vi "Proyecto 1.vi"() -> ()   [LabVIEW 2020]
uses:
  <vilib>/numeric/Random Number (Range) U64.vi
  <vilib>/numeric/Random Number (Range) I64.vi
  <vilib>/numeric/sub_Random U32.vi
panel:
  out "enum5":i16
  out "sum":i16
  out "Enum 4":enum8{"0", "1", "2", "3", "4", "5", "6"}(ring)
  out "Enum 3":enum8{"1", "2", "3", "4", "5", "6"}(ring)
  out "DiskAcum":i64
  out "TAP 2":string[][](array[string])
  out "Size":string[](array[string])
  out "MemoryMap":string[](array[string])
  out "TAP":string[][](array[string])
  out "Waiting 2":string[](array[string])
  out "Printing 2":string
  in  "FrameSize":i8(slide) step=1 scale=4.0..64.0
  in  "RAMSize":i64(slide) min=0 step=4 scale=32.0..256.0
  in  "ProbMemoria":i8(slide) step=10 scale=0.0..100.0
  out "element":string
  out "ID":string[](array[string])
  out "QuantumAcum":i64
  out "Enum 2":enum16{"1", "2", "3"}(ring)
  out "Tiempo de impresión":string[](array[string])
  out "Hora uso i/o":string[](array[string])
  out "Uso de impresora":string[](array[string])
  out "Duración":string[](array[string])
  out "Enum":enum16{"1", "2", "3"}(ring)=enum."3"
  out "Hora de llegada":string[](array[string])
  out "PCB":string[][](array[string])
  out "Terminated":string[](array[string])
  out "Waiting":string[](array[string])
  out "Ready":string[](array[string])
  out "New":string[](array[string])
  out "Printing":string
  out "Running":string
  in  "Delay":i32(slide)
  out "Clock":i32
  in  "play/pause":bool
  in  "DurImpresora":i8(slide) step=10 scale=10.0..80.0
  in  "ProbImpresora":i8(slide) step=10 scale=0.0..100.0
  in  "DurProceso":i8(slide) step=10 scale=5.0..100.0
  in  "Quantum":i8(slide) step=10 scale=0.0..20.0
  in  "stop":bool
  in  "ProbProceso":i8(slide) step=10 scale=0.0..100.0
  # "RELOJ"
  # "PROCESS & MEMORY MANAGER"
  # "LENTO"
  # "NORMAL"
  # "RÁPIDO"
  # "QUANTUM"
  # "NEW"
  # "READY"
  # "RUNNING"
  # "WAITING I/0"
  # "USING I/0"
  # "WAITING DISK"
  # "USING DISK"
  # "TERMINATED"
  # "MEMORY MAP"
  # "0\n1\n2\n3\n4\n5\n6\n7\n8\n9\n10\n11\n12\n13\n14\n15\n16\n17\n18\n19\n20\n21\n22\n23\n24"
  # "PROB GENERAR PROCESO"
  # "DURACIÓN PROCESO"
  # "PROB USO I/0"
  # "TAP"
  # "PROCESS CONTROL BLOCK"
  # "e"
  # "d"
  # "H I/O"
  # "ID"
  # "a"
  # "b"
  # "c"
  # "f"
  # "I/O"
  # "T I/O"
  # "SIZE (KB)"
  # "ID"
  # "AT"
  # "DUR"
  # "ACUM"
  # "DURACIÓN I/0"
  # "PROB USO MEMORIA"
  # "RAM SIZE"
  # "FRAME SIZE"
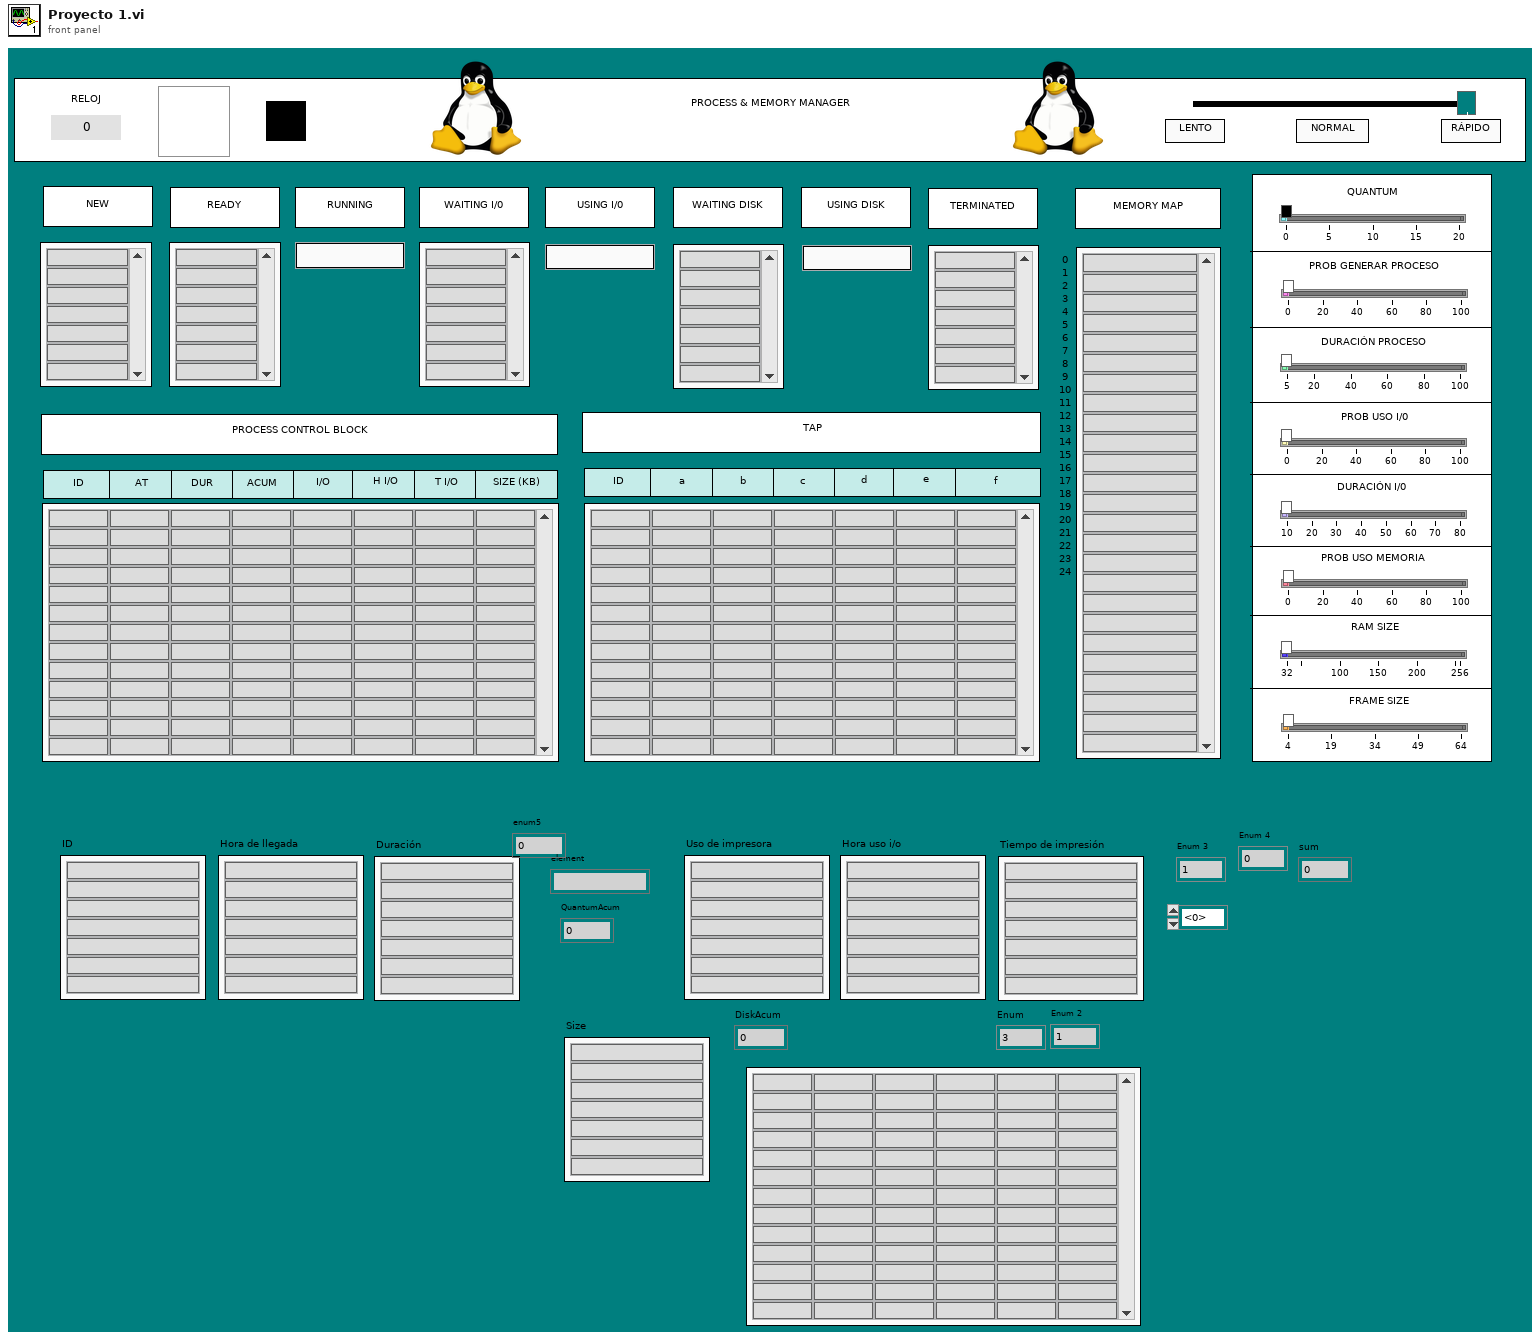
[diagram p1: front panel]
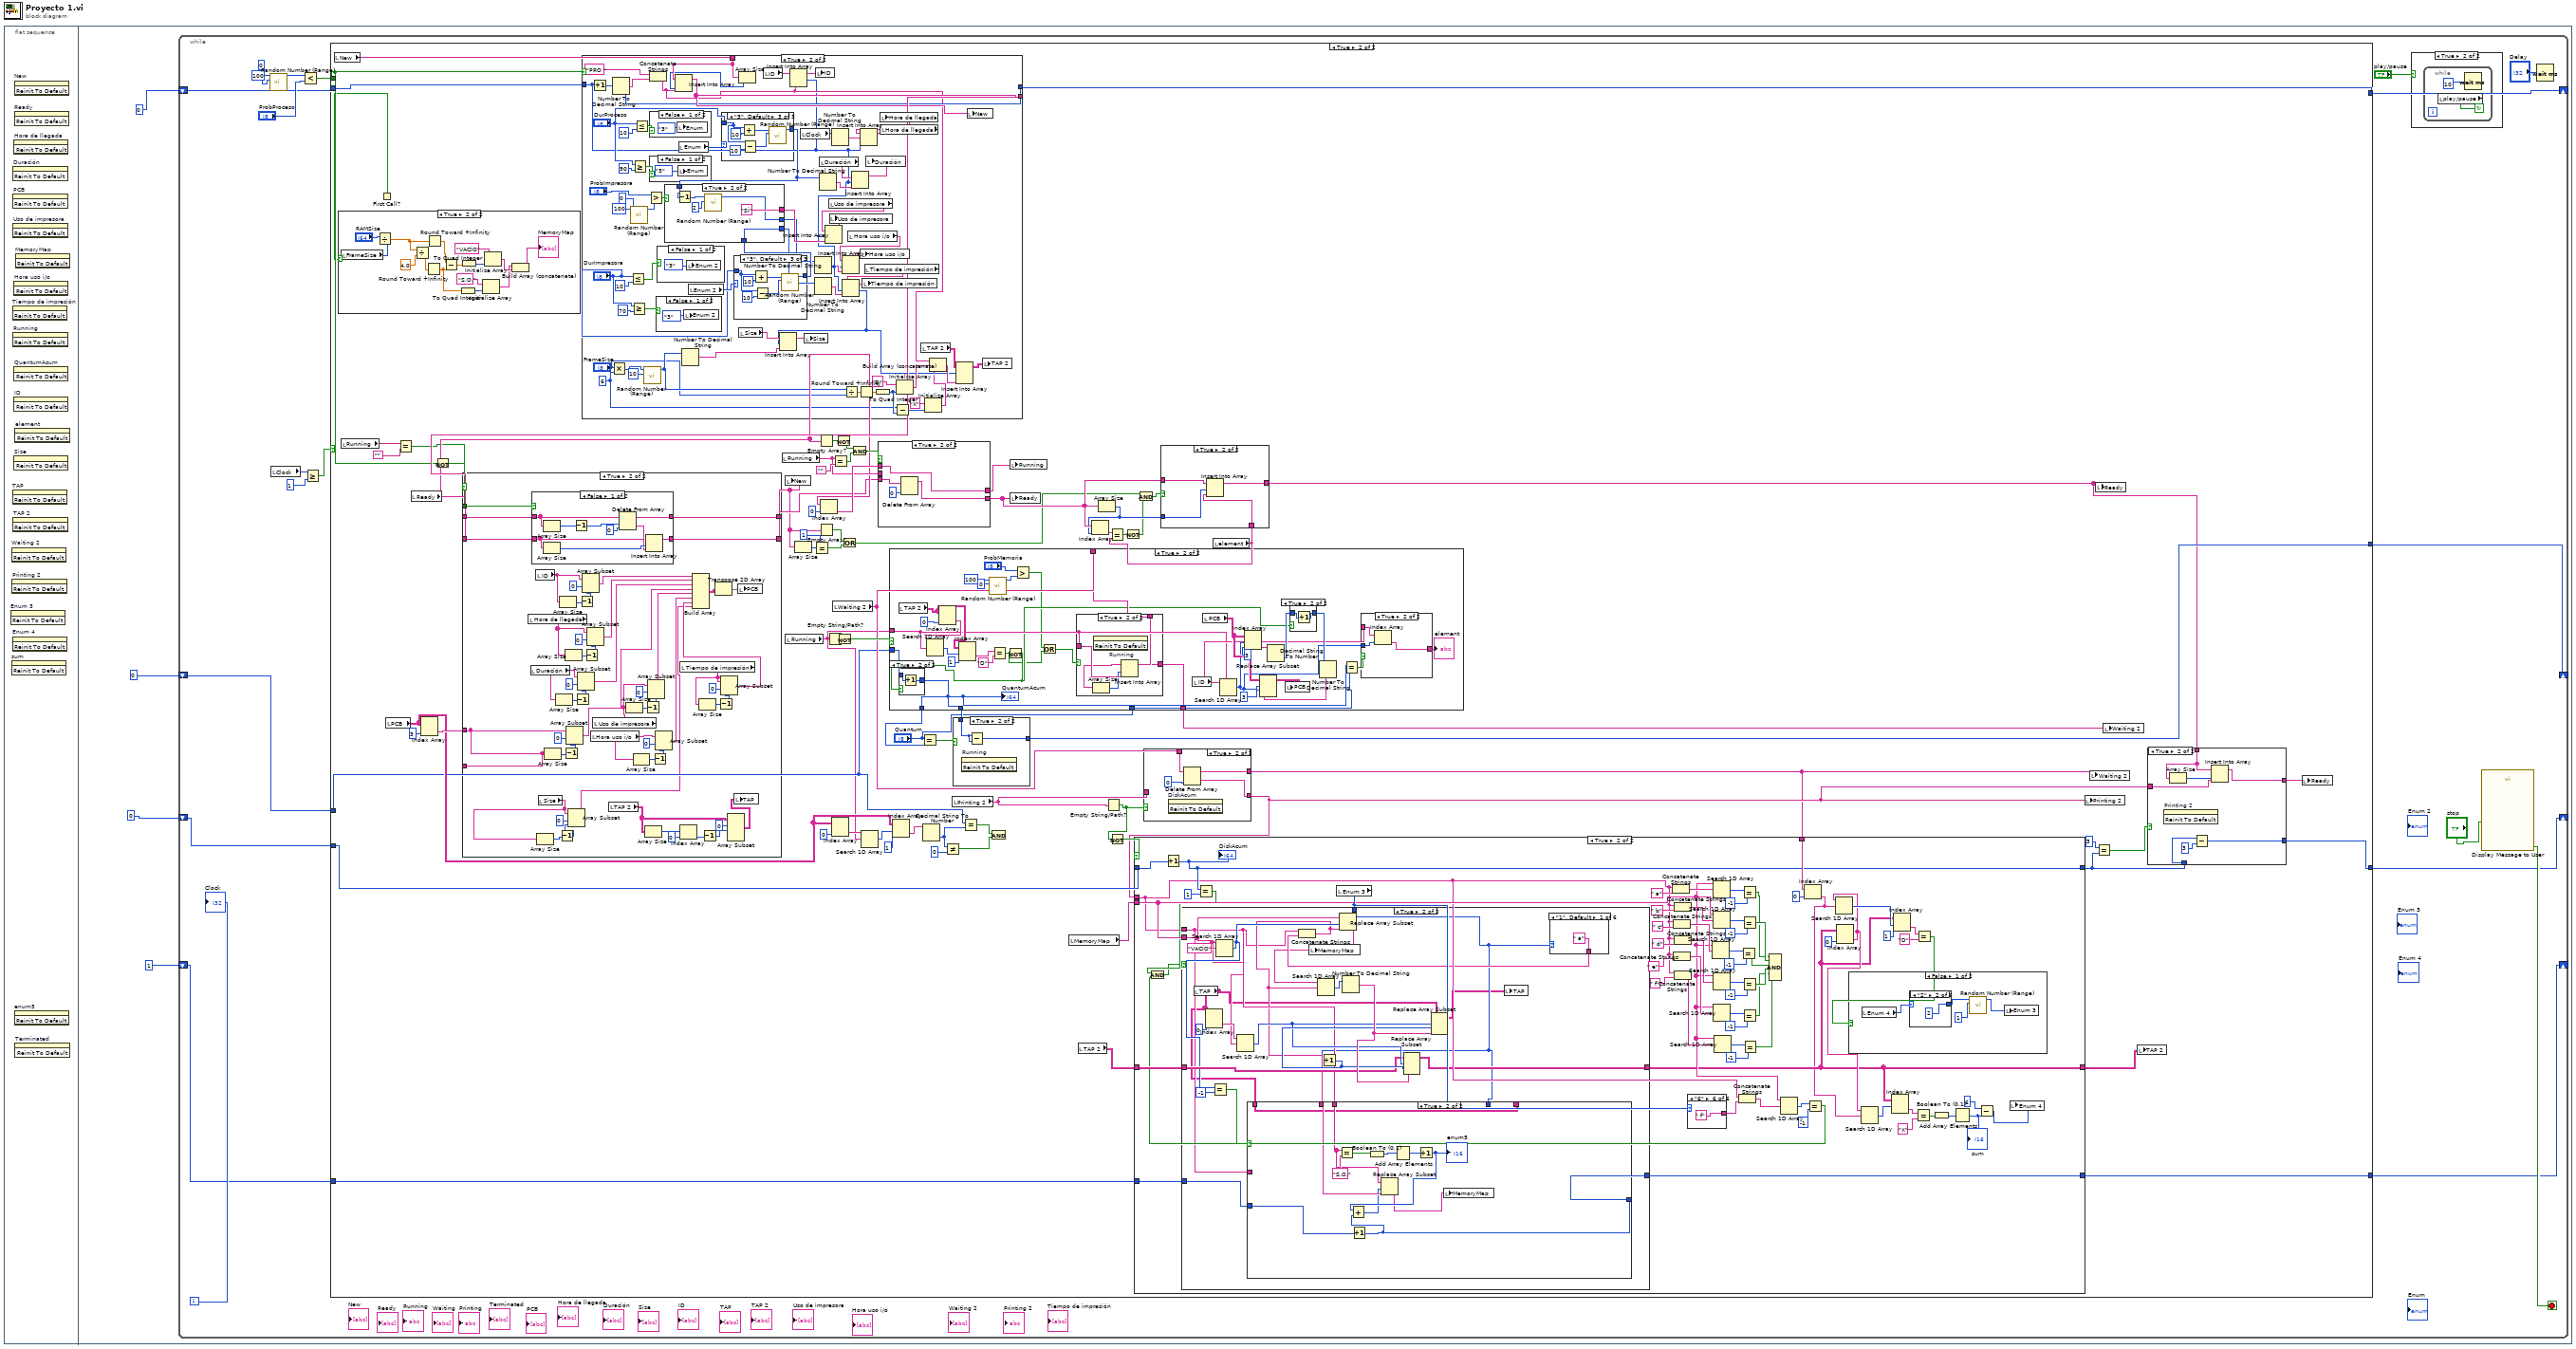
[diagram p0: block diagram]
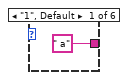
[diagram p6: hidden frame]
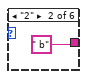
[diagram p7: hidden frame]
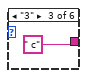
[diagram p8: hidden frame]
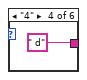
[diagram p9: hidden frame]
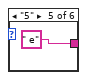
[diagram p10: hidden frame]
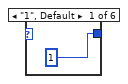
[diagram p11: hidden frame]
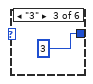
[diagram p12: hidden frame]
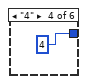
[diagram p13: hidden frame]
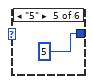
[diagram p14: hidden frame]
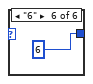
[diagram p15: hidden frame]
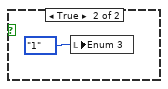
[diagram p16: hidden frame]
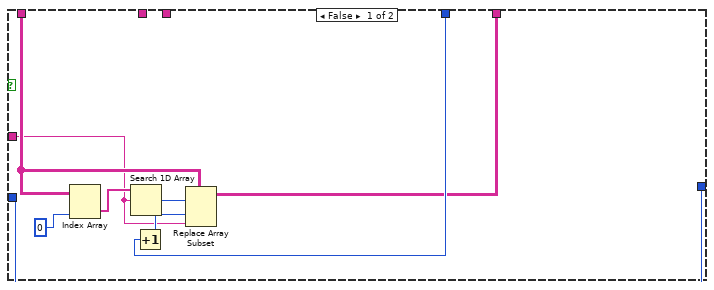
[diagram p18: hidden frame]
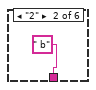
[diagram p19: hidden frame]
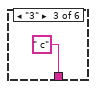
[diagram p20: hidden frame]
diagram:
  n1 = flat-sequence {
    frame #0 {
      n2 = invoke on="Enum 3" class="Enum (strict)" method="Reinit To Default"() -> ()  [unwired: 3 in, 3 out]
      n3 = invoke on="Waiting 2" class="Arr (strict)" method="Reinit To Default"() -> ()  [unwired: 3 in, 3 out]
      n4 = invoke on="sum" class="DigNum (strict)" method="Reinit To Default"() -> ()  [unwired: 3 in, 3 out]
      n5 = invoke on="Printing 2" class="Str" method="Reinit To Default"() -> ()  [unwired: 3 in, 3 out]
      n6 = invoke on="Tiempo de impresión" class="Arr (strict)" method="Reinit To Default"() -> ()  [unwired: 3 in, 3 out]
      n7 = invoke on="TAP" class="Arr (strict)" method="Reinit To Default"() -> ()  [unwired: 3 in, 3 out]
      n8 = invoke on="Enum 4" class="Enum (strict)" method="Reinit To Default"() -> ()  [unwired: 3 in, 3 out]
      n9 = invoke on="Duración" class="Arr (strict)" method="Reinit To Default"() -> ()  [unwired: 3 in, 3 out]
      n10 = invoke on="PCB" class="Arr (strict)" method="Reinit To Default"() -> ()  [unwired: 3 in, 3 out]
      n11 = invoke on="Uso de impresora" class="Arr (strict)" method="Reinit To Default"() -> ()  [unwired: 3 in, 3 out]
      n12 = invoke on="Running" class="Str" method="Reinit To Default"() -> ()  [unwired: 3 in, 3 out]
      n13 = invoke on="TAP 2" class="Arr (strict)" method="Reinit To Default"() -> ()  [unwired: 3 in, 3 out]
      n14 = invoke on="Hora de llegada" class="Arr (strict)" method="Reinit To Default"() -> ()  [unwired: 3 in, 3 out]
      n15 = invoke on="Hora uso i/o" class="Arr (strict)" method="Reinit To Default"() -> ()  [unwired: 3 in, 3 out]
      n16 = invoke on="QuantumAcum" class="DigNum (strict)" method="Reinit To Default"() -> ()  [unwired: 3 in, 3 out]
      n17 = invoke on="ID" class="Arr (strict)" method="Reinit To Default"() -> ()  [unwired: 3 in, 3 out]
      n18 = invoke on="Size" class="Arr (strict)" method="Reinit To Default"() -> ()  [unwired: 3 in, 3 out]
      n19 = invoke on="New" class="Arr (strict)" method="Reinit To Default"() -> ()  [unwired: 3 in, 3 out]
      n20 = invoke on="Ready" class="Arr (strict)" method="Reinit To Default"() -> ()  [unwired: 3 in, 3 out]
      n21 = invoke on="enum5" class="DigNum (strict)" method="Reinit To Default"() -> ()  [unwired: 3 in, 3 out]
      n22 = invoke on="element" class="Str" method="Reinit To Default"() -> ()  [unwired: 3 in, 3 out]
      n23 = invoke on="Terminated" class="Arr (strict)" method="Reinit To Default"() -> ()  [unwired: 3 in, 3 out]
      n24 = invoke on="MemoryMap" class="Arr (strict)" method="Reinit To Default"() -> ()  [unwired: 3 in, 3 out]
    }
    frame #1 {
      n25 = while {
        shift-right: [w15] -> _
        shift-left: 0 -> [w11]
        shift-right: [w9] -> _
        shift-left: i64 0 ("QuantumAcum") -> [w10]
        shift-right: [w7] -> _
        shift-left: i64 0 ("QuantumAcum") -> [w8]
        shift-right: [w6] -> _
        shift-left: i16 1 ("enum5") -> [w5]
        i -> [w22]
        stop <- w25 stop-if-true
        n26 = call-poly <vilib>:"Random Number (Range).vi"("lower bound (0)"=u64 0, "upper bound (100)"=u64 100) -> ("number"=w17:u64)  [unwired: 9 in]
        n27 = local read "Clock"() -> (w14:i32)
        n28 = Less?(x=w17, y="ProbProceso") -> (x < y?=w16:bool)
        n29 = Greater Or Equal?(x=w14, y=1) -> (x >= y?=w12:bool)
        n30 = case shown="True" w12 {
          tunnel: w11 -> [w29 w103]
          tunnel: w16 -> [_ w97]
          tunnel: [w29 w102] -> w15
          tunnel: w10 -> [w28 w35]
          tunnel: [w28 w80] -> w9
          tunnel: w8 -> [w27 w58]
          tunnel: [w27 w48] -> w7
          tunnel: w5 -> [w26 w43]
          tunnel: [w26 w42] -> w6
          frame False {
          }
          frame True {
            n31 = local read "New"() -> (w100:string[])
            n32 = local read "Running"() -> (w101:string)
            n33 = First Call?() -> (First Call?: T/F=w54:bool)
            n34 = case shown="True" w54 {
              frame False {
              }
              frame True {
                n35 = local read "FrameSize"() -> (w117:i8)
                n36 = Divide(x="RAMSize", y=w117) -> (x/y=w115:dbl)
                n37 = Divide(x=w115, y=4.0) -> (x/y=w113:dbl)
                n38 = Round Toward +Infinity(x=w113) -> (ceil(x): smallest int >= x=w109:dbl)
                n39 = Round Toward +Infinity(x=w115) -> (ceil(x): smallest int >= x=w114:dbl)
                n40 = Subtract(x=w114, y=w109) -> (x-y=w112:dbl)
                n41 = To Quad Integer(1:w109) -> (0:w108:i64)
                n42 = To Quad Integer(1:w112) -> (0:w111:i64)
                n43 = Initialize Array("S.O." ("element"), w108) -> (w105:string[])
                n44 = Initialize Array("VACÍO" ("element"), w111) -> (w106:string[])
                n45 = Build Array (concatenate)(w105, w106) -> (→"MemoryMap":string[])
              }
            }
            n46 = local read "PCB"() -> (w39:string[][])
            n47 = Equal?(x=w101, y="") -> (x = y?=w68:bool)
            n48 = local read "Ready"() -> (w82:string[])
            n49 = Index Array(array=w39, index (col)=3 ("disabled index (col)")) -> (element=w76:string[])  [unwired: 1 in]
            n50 = Not(x=w97) -> (.not. x?=w98:bool)
            n51 = case shown="True" w97 {
              tunnel: w103 -> [w409 w417]
              tunnel: [w409 w433] -> w102
              tunnel: w100 -> [w408 w437]
              tunnel: [w408 w436] -> w99
              frame False {
              }
              frame True {
                w413 = i8 6 ("y")
                n52 = Increment(x=w417) -> (x+1=w433:i32)
                n53 = Multiply(x="FrameSize", y=w413) -> (x*y=w430:i8)
                n54 = Number To Decimal String(number=w433) -> (decimal integer string=w474:string)  [unwired: 1 in]
                n55 = Less Or Equal?(x="DurImpresora", y=i8 10) -> (x <= y?=w450:bool)
                n56 = call-poly <vilib>:"Random Number (Range).vi"("lower bound (0)"=u64 0, "upper bound (100)"=u64 100) -> ("number"=w458:u64)  [unwired: 9 in]
                n57 = Greater Or Equal?(x="DurImpresora", y=i8 70) -> (x >= y?=w448:bool)
                n58 = Greater Or Equal?(x="DurProceso", y=i8 90) -> (x >= y?=w466:bool)
                n59 = Less Or Equal?(x="DurProceso", y=i8 10) -> (x <= y?=w468:bool)
                n60 = call-poly <vilib>:"Random Number (Range).vi"("lower bound (0)"=u64 10, "upper bound (100)"=w430) -> ("number"=w422:u64)  [unwired: 9 in]
                n61 = Greater?(x="ProbImpresora", y=w458) -> (0:w456:bool)
                n62 = Concatenate Strings("PRO ", w474) -> (w420:string)
                n63 = case shown="False" w468 {
                  frame False {
                    n64 = local write "Enum"(enum16{"1", "2", "3"}."3") -> ()
                  }
                  frame True {
                    n65 = local write "Enum"(enum16{"1", "2", "3"}."1" ("Enum")) -> ()
                  }
                }
                n66 = case shown="False" w466 {
                  frame False {
                    n67 = local write "Enum"(enum16{"1", "2", "3"}."3") -> ()
                  }
                  frame True {
                    n68 = local write "Enum"(enum16{"1", "2", "3"}."2") -> ()
                  }
                }
                n69 = case shown="False" w448 {
                  frame False {
                    n70 = local write "Enum 2"(enum16{"1", "2", "3"}."3") -> ()
                  }
                  frame True {
                    n71 = local write "Enum 2"(enum16{"1", "2", "3"}."2") -> ()
                  }
                }
                n72 = case shown="False" w450 {
                  frame False {
                    n73 = local write "Enum 2"(enum16{"1", "2", "3"}."3") -> ()
                  }
                  frame True {
                    n74 = local write "Enum 2"(enum16{"1", "2", "3"}."1") -> ()
                  }
                }
                n75 = local read "Enum"() -> (w465:enum16{"1", "2", "3"})
                n76 = Number To Decimal String(number=w422) -> (decimal integer string=w425:string)  [unwired: 1 in]
                n77 = local read "Enum 2"() -> (w447:enum16{"1", "2", "3"})
                n78 = case shown="\"3\", Default" w465 {
                  tunnel: "DurProceso" -> [w507 w511 w518]
                  tunnel: [w505 w510 w515] -> w452
                  frame "1" {
                    n79 = Add(x=w507, y=i8 10) -> (x+y=w509:i8)
                    n80 = call-poly <vilib>:"Random Number (Range).vi"("lower bound (0)"=u64 1, "upper bound (100)"=w509) -> ("number"=w505:u64)  [unwired: 9 in]
                  }
                  frame "2" {
                    n81 = Subtract(x=w511, y=i8 10) -> (x-y=w514:i8)
                    n82 = call-poly <vilib>:"Random Number (Range).vi"("lower bound (0)"=w514, "upper bound (100)"=u64 100 ("lower bound (0)")) -> ("number"=w510:u64)  [unwired: 9 in]
                  }
                  frame "3", Default {
                    n83 = Add(x=w518, y=i8 10) -> (x+y=w519:i8)
                    n84 = Subtract(x=w518, y=i8 10) -> (x-y=w516:i8)
                    n85 = call-poly <vilib>:"Random Number (Range).vi"("lower bound (-100)"=w516, "upper bound (100)"=w519) -> ("number"=w515:i64)  [unwired: 9 in]
                  }
                }
                n86 = case shown="\"3\", Default" w447 {
                  tunnel: "DurImpresora" -> [w478 w482 w487]
                  tunnel: [w476 w481 w486] -> w445
                  frame "1" {
                    n87 = Add(x=w478, y=i8 10) -> (x+y=w477:i8)
                    n88 = call-poly <vilib>:"Random Number (Range).vi"("lower bound (0)"=u64 1, "upper bound (100)"=w477) -> ("number"=w476:u64)  [unwired: 9 in]
                  }
                  frame "2" {
                    n89 = Subtract(x=w482, y=i8 10) -> (x-y=w485:i8)
                    n90 = call-poly <vilib>:"Random Number (Range).vi"("lower bound (0)"=w485, "upper bound (100)"=u64 80 ("lower bound (0)")) -> ("number"=w481:u64)  [unwired: 9 in]
                  }
                  frame "3", Default {
                    n91 = Add(x=w487, y=i8 10) -> (x+y=w490:i8)
                    n92 = Subtract(x=w487, y=i8 10) -> (x-y=w488:i8)
                    n93 = call-poly <vilib>:"Random Number (Range).vi"("lower bound (-100)"=w488, "upper bound (100)"=w490) -> ("number"=w486:i64)  [unwired: 9 in]
                  }
                }
                n94 = case shown="True" w456 {
                  tunnel: ["NO" "SÍ"] -> w455
                  tunnel: w452 -> [_ w503]
                  tunnel: [u64 0 ("number") w501] -> w444
                  tunnel: [u64 0 ("number") w500] -> w441
                  tunnel: w445 -> [_ w500]
                  frame False {
                  }
                  frame True {
                    n95 = Decrement(x=w503) -> (x-1=w502:u64)
                    n96 = call-poly <vilib>:"Random Number (Range).vi"("lower bound (0)"=u64 2, "upper bound (100)"=w502) -> ("number"=w501:u64)  [unwired: 9 in]
                  }
                }
                n97 = Array Size(array=w437) -> (size(s)=w432:i32)
                n98 = Insert Into Array(array=w437, index=w432, new element=w420) -> (w436:string[])
                n99 = local read "Size"() -> (w424:string[])
                n100 = local read "ID"() -> (w435:string[])
                n101 = Insert Into Array(array=w424, index=w417, new element=w425) -> (w429:string[])
                n102 = Insert Into Array(array=w435, index=w417, new element=w420) -> (w434:string[])
                n103 = local read "Clock"() -> (w473:i32)
                n104 = local write "Size"(w429) -> ()
                n105 = Number To Decimal String(number=w444) -> (decimal integer string=w440:string)  [unwired: 1 in]
                n106 = Number To Decimal String(number=w441) -> (decimal integer string=w423:string)  [unwired: 1 in]
                n107 = local write "ID"(w434) -> ()
                n108 = Number To Decimal String(number=w452) -> (decimal integer string=w463:string)  [unwired: 1 in]
                n109 = local read "Duración"() -> (w462:string[])
                n110 = local read "Uso de impresora"() -> (w453:string[])
                n111 = Insert Into Array(array=w453, index=w417, new element=w455) -> (w454:string[])
                n112 = local write "Uso de impresora"(w454) -> ()
                n113 = Number To Decimal String(number=w473) -> (decimal integer string=w472:string)  [unwired: 1 in]
                n114 = Divide(x=w422, y="FrameSize") -> (x/y=w427:dbl)
                n115 = local read "Hora uso i/o"() -> (w443:string[])
                n116 = Insert Into Array(array=w443, index=w417, new element=w440) -> (w442:string[])
                n117 = Insert Into Array(array=w462, index=w417, new element=w463) -> (w461:string[])
                n118 = Round Toward +Infinity(x=w427) -> (ceil(x): smallest int >= x=w428:dbl)
                n119 = local write "Hora uso i/o"(w442) -> ()
                n120 = local read "Tiempo de impresión"() -> (w439:string[])
                n121 = Insert Into Array(array=w439, index=w417, new element=w423) -> (w438:string[])
                n122 = local write "Tiempo de impresión"(w438) -> ()
                n123 = local write "Duración"(w461) -> ()
                n124 = To Quad Integer(1:w428) -> (0:w414:i64)
                n125 = local read "Hora de llegada"() -> (w471:string[])
                n126 = Insert Into Array(array=w471, index=w417, new element=w472) -> (w470:string[])
                n127 = local write "Hora de llegada"(w470) -> ()
                n128 = Subtract(x=w413, y=w414) -> (x-y=w412:i64)
                n129 = Initialize Array("D", w414) -> (w421:string[])
                n130 = local read "TAP 2"() -> (w416:string[][])
                n131 = Initialize Array("X" ("element"), w412) -> (w410:string[])
                n132 = Build Array (concatenate)(w420, w421, w410) -> (w418:string[])
                n133 = Insert Into Array(array=w416, index (row)=w417, new element=w418) -> (w415:string[][])  [unwired: 1 in]
                n134 = local write "New"(w436) -> ()
                n135 = local write "TAP 2"(w415) -> ()
              }
            }
            n136 = case shown="True" w68 {
              tunnel: w99 -> [w335 w390]
              tunnel: w82 -> [w336 w389]
              tunnel: [w336 w384] -> w78
              tunnel: w98 -> [_ w388]
              tunnel: [w335 w387] -> w67
              tunnel: w76 -> [w334 w350]
              tunnel: [w334 w350] -> _
              frame False {
              }
              frame True {
                n137 = local read "Hora de llegada"() -> (w376:string[])
                n138 = local read "Duración"() -> (w371:string[])
                n139 = case shown="False" w388 {
                  tunnel: w390 -> [w396 w407]
                  tunnel: w389 -> [w395 w406]
                  tunnel: [w394 w405] -> w384
                  tunnel: [w391 w400] -> w387
                  frame False {
                    n140 = Array Size(array=w396) -> (size(s)=w393:i32)
                    n141 = Array Size(array=w395) -> (size(s)=w399:i32)
                    n142 = Decrement(x=w393) -> (x-1=w392:i32)
                    n143 = Delete From Array(array=w396, length=w392, index=0) -> (deleted portion=w398:string[], array with subset deleted=w391:string[])
                    n144 = Insert Into Array(array=w395, index=w399, new element=w398) -> (w394:string[])
                  }
                  frame True {
                    n145 = Array Size(array=w407) -> (size(s)=w404:i32)
                    n146 = Array Size(array=w406) -> (size(s)=w402:i32)
                    n147 = Delete From Array(array=w407, length=w404, index=0) -> (deleted portion=w403:string[], array with subset deleted=w400:string[])
                    n148 = Insert Into Array(array=w406, index=w402, new element=w403) -> (w405:string[])
                  }
                }
                n149 = local read "ID"() -> (w382:string[])
                n150 = local read "Size"() -> (w344:string[])
                n151 = Array Size(array=w344) -> (size(s)=w345:i32)
                n152 = Array Size(array=w350) -> (size(s)=w368:i32)
                n153 = Array Size(array=w371) -> (size(s)=w373:i32)
                n154 = Decrement(x=w345) -> (x-1=w349:i32)
                n155 = Array Size(array=w382) -> (size(s)=w381:i32)
                n156 = Decrement(x=w368) -> (x-1=w367:i32)
                n157 = Array Size(array=w376) -> (size(s)=w378:i32)
                n158 = Array Subset(array=w350, index=0, length=w367) -> (w351:string[])
                n159 = Array Subset(array=w344, index=0, length=w349) -> (w346:string[])
                n160 = Decrement(x=w373) -> (x-1=w372:i32)
                n161 = Array Subset(array=w371, index=0, length=w372) -> (w370:string[])
                n162 = Decrement(x=w381) -> (x-1=w380:i32)
                n163 = Array Subset(array=w382, index=0, length=w380) -> (w347:string[])
                n164 = Decrement(x=w378) -> (x-1=w377:i32)
                n165 = Array Subset(array=w376, index=0, length=w377) -> (w375:string[])
                n166 = local read "Hora uso i/o"() -> (w358:string[])
                n167 = local read "Uso de impresora"() -> (w363:string[])
                n168 = local read "TAP 2"() -> (w338:string[][])
                n169 = Array Size(array=w363) -> (size(s)=w365:i32)
                n170 = Array Size(array=w358) -> (size(s)=w360:i32)
                n171 = Decrement(x=w365) -> (x-1=w364:i32)
                n172 = Array Size(array=w338) -> (size(s)=w343:i32[])
                n173 = Array Subset(array=w363, index=0, length=w364) -> (w362:string[])
                n174 = Decrement(x=w360) -> (x-1=w359:i32)
                n175 = Array Subset(array=w358, index=0, length=w359) -> (w357:string[])
                n176 = Index Array(array=w343, index=0) -> (element=w341:i32)
                n177 = local read "Tiempo de impresión"() -> (w353:string[])
                n178 = Array Size(array=w353) -> (size(s)=w355:i32)
                n179 = Decrement(x=w341) -> (x-1=w340:i32)
                n180 = Decrement(x=w355) -> (x-1=w354:i32)
                n181 = Array Subset(array=w353, index=0, length=w354) -> (w352:string[])
                n182 = Build Array(w347, w375, w370, w351, w362, w357, w352, w346) -> (w385:string[][])
                n183 = Transpose 2D Array(2D array=w385) -> (transposed array=w386:string[][])
                n184 = Array Subset(array=w338, index (row)=0 ("index"), length (row)=w340) -> (w337:string[][])  [unwired: 2 in]
                n185 = local write "TAP"(w337) -> ()
                n186 = local write "PCB"(w386) -> ()
              }
            }
            n187 = local read "Running"() -> (w83:string)
            n188 = local write "New"(w67) -> ()
            n189 = local read "Running"() -> (w34:string)
            n190 = Array Size(array=w67) -> (size(s)=w66:i32)
            n191 = Equal?(x=w66, y=1) -> (x = y?=w63:bool)
            n192 = Empty Array?(array=w82) -> (empty?=w92:bool)
            n193 = Empty Array?(array=w67) -> (empty?=w64:bool)
            n194 = Index Array(array=w82, index=0) -> (element=w93:string)
            n195 = Empty String/Path?(string/path=w34) -> (empty?=w88:bool)
            n196 = Equal?(x=w83, y="") -> (x = y?=w90:bool)
            n197 = Index Array(array=w39, index (col)=0 ("disabled index (col)")) -> (element=w40:string[])  [unwired: 1 in]
            n198 = local read "Waiting 2"() -> (w55:string[])
            n199 = Not(x=w92) -> (.not. x?=w91:bool)
            n200 = Not(x=w88) -> (.not. x?=w87:bool)
            n201 = Or(x=w64, y=w63) -> (x .or. y?=w62:bool)
            n202 = And(x=w91, y=w90) -> (x .and. y?=w89:bool)
            n203 = Search 1D Array(1D array=w40, element=w34) -> (index of element=w38:i32)  [unwired: 1 in]
            n204 = case shown="True" w89 {
              tunnel: w93 -> [_ w330]
              tunnel: w78 -> [w329 w333]
              tunnel: [w329 w331] -> w75
              tunnel: [w328 w330] -> w84
              tunnel: w83 -> [w328 _]
              frame False {
              }
              frame True {
                n205 = Delete From Array(array=w333, index=0) -> (array with subset deleted=w331:string[])  [unwired: 1 in, 1 out]
              }
            }
            n206 = case shown="True" w87 {
              tunnel: w35 -> [w279 w312]
              tunnel: [w279 w304] -> w81
              tunnel: [w279 w304] -> w85
              tunnel: w34 -> [_ w290]
              tunnel: "Quantum" -> [_ w303]
              tunnel: w55 -> [w278 w289]
              tunnel: [w278 w288] -> w61
              frame False {
              }
              frame True {
                n207 = local read "TAP 2"() -> (w295:string[][])
                n208 = Index Array(array=w295, index (col)=0 ("disabled index (col)")) -> (element=w296:string[])  [unwired: 1 in]
                n209 = Search 1D Array(1D array=w296, element=w290) -> (index of element=w294:i32)  [unwired: 1 in]
                n210 = Index Array(array=w295, index (row)=w294, index (col)=1 ("disabled index (col)")) -> (element=w292:string)
                n211 = call-poly <vilib>:"Random Number (Range).vi"("lower bound (0)"=u64 0, "upper bound (100)"=u64 100) -> ("number"=w284:u64)  [unwired: 9 in]
                n212 = Equal?(x=w292, y="D") -> (x = y?=w282:bool)
                n213 = Not(x=w282) -> (.not. x?=w287:bool)
                n214 = case shown="True" w287 {
                  tunnel: w312 -> [w321 w323]
                  tunnel: [w321 w322] -> w304
                  frame False {
                  }
                  frame True {
                    n215 = Increment(x=w323) -> (x+1=w322:i64)
                  }
                }
                "QuantumAcum" <- w304
                n216 = Greater?(x="ProbMemoria", y=w284) -> (0:w280:bool)
                n217 = Or(x=w280, y=w282) -> (x .or. y?=w281:bool)
                n218 = case shown="True" w281 {
                  tunnel: w290 -> [_ w320]
                  tunnel: w289 -> [w316 w319]
                  tunnel: [w316 w317] -> w288
                  frame False {
                  }
                  frame True {
                    n219 = Array Size(array=w319) -> (size(s)=w318:i32)
                    n220 = invoke on="Running" class="Str" method="Reinit To Default"() -> ()  [unwired: 3 in, 3 out]
                    n221 = Insert Into Array(array=w319, index=w318, new element=w320) -> (w317:string[])
                  }
                }
                n222 = local read "ID"() -> (w299:string[])
                n223 = local read "PCB"() -> (w305:string[][])
                n224 = Search 1D Array(1D array=w299, element=w290) -> (index of element=w300:i32)  [unwired: 1 in]
                n225 = Index Array(array=w305, index (row)=w300, index (col)=3 ("disabled index (col)")) -> (element=w308:string)
                n226 = Decimal String To Number(string=w308) -> (number=w310:i32)  [unwired: 2 in, 1 out]
                n227 = case shown="True" w287 {
                  tunnel: [w313 w315] -> w311
                  tunnel: w310 -> [w313 w314]
                  frame False {
                  }
                  frame True {
                    n228 = Increment(x=w314) -> (x+1=w315:i32)
                  }
                }
                n229 = Number To Decimal String(number=w311) -> (decimal integer string=w301:string)  [unwired: 1 in]
                n230 = Replace Array Subset(array=w305, new element=w301, index (row)=w300, index (col)=3 ("disabled index (col)")) -> (w307:string[][])
                n231 = local write "PCB"(w307) -> ()
                n232 = Equal?(x=w304, y=w303) -> (x = y?=w302:bool)
                n233 = case shown="True" w302 {
                  tunnel: w300 -> [_ w327]
                  tunnel: w299 -> [_ w326]
                  tunnel: ["" w325] -> w298
                  frame False {
                  }
                  frame True {
                    n234 = Index Array(array=w326, index=w327) -> (element=w325:string)
                  }
                }
                "element" <- w298
              }
            }
            n235 = Index Array(array=w39, index (row)=w38, index (col)=1 ("disabled index (col)")) -> (element=w36:string)
            n236 = Equal?(x="Quantum", y=w85) -> (x = y?=w86:bool)
            n237 = Decimal String To Number(string=w36) -> (number=w33:i32)  [unwired: 2 in, 1 out]
            n238 = Not Equal?(x=w33, y=0) -> (x != y?=w30:bool)
            n239 = local read "Printing 2"() -> (w52:string)
            n240 = case shown="True" w86 {
              tunnel: w81 -> [w275 w277]
              tunnel: [w275 w276] -> w80
              frame False {
              }
              frame True {
                n241 = invoke on="Running" class="Str" method="Reinit To Default"() -> ()  [unwired: 3 in, 3 out]
                n242 = Subtract(x=w277, y=w277) -> (x-y=w276:i64)
              }
            }
            n243 = Equal?(x=w35, y=w33) -> (x = y?=w31:bool)
            n244 = And(x=w31, y=w30) -> ()  [unwired: 1 out]
            n245 = local write "Running"(w84) -> ()
            n246 = local write "Ready"(w75) -> ()
            n247 = local read "MemoryMap"() -> (w53:string[])
            n248 = local read "TAP 2"() -> (w50:string[][])
            n249 = Array Size(array=w75) -> (size(s)=w74:i32)
            n250 = Index Array(array=w75, index=w74) -> (element=w73:string)
            n251 = Empty String/Path?(string/path=w52) -> (empty?=w60:bool)
            n252 = Not(x=w60) -> (.not. x?=w59:bool)
            n253 = case shown="True" w60 {
              tunnel: w55 -> [w264 w268]
              tunnel: [w265 w266] -> w46
              tunnel: w52 -> [w265 _]
              tunnel: [w264 w267] -> w44
              frame False {
              }
              frame True {
                n254 = invoke on="DiskAcum" class="DigNum (strict)" method="Reinit To Default"() -> ()  [unwired: 3 in, 3 out]
                n255 = Delete From Array(array=w268, index=0) -> (deleted portion=w266:string, array with subset deleted=w267:string[])  [unwired: 1 in]
              }
            }
            n256 = case shown="True" w59 {
              tunnel: w58 -> [w130 w195]
              tunnel: [w130 w150] -> w49
              tunnel: w53 -> [_ w153]
              tunnel: w46 -> [_ w137]
              tunnel: [w129 w143] -> w51
              tunnel: w50 -> [w129 w166]
              tunnel: w44 -> [_ w159]
              tunnel: w43 -> [w128 w132]
              tunnel: [w128 w131] -> w42
              frame False {
              }
              frame True {
                n257 = Increment(x=w195) -> (x+1=w150:i64)
                "DiskAcum" <- w150
                n258 = Equal?(x=w150, y=i64 1) -> (x = y?=w147:bool)
                n259 = local read "Enum 3"() -> (w156:enum8{"1", "2", "3", "4", "5", "6"})
                n260 = Concatenate Strings(w137, " a") -> (w186:string)
                n261 = Concatenate Strings(w137, " c") -> (w180:string)
                n262 = Concatenate Strings(w137, " e") -> (w174:string)
                n263 = Concatenate Strings(w137, " b") -> (w183:string)
                n264 = Concatenate Strings(w137, " d") -> (w177:string)
                n265 = Concatenate Strings(w137, " f") -> (w145:string)
                n266 = case shown="\"6\"" w156 {
                  tunnel: [" a" " b" " c" " d" " e" " f"] -> w155
                  frame "1", Default {
                  }
                  frame "2" {
                  }
                  frame "3" {
                  }
                  frame "4" {
                  }
                  frame "5" {
                  }
                  frame "6" {
                  }
                }
                n267 = Search 1D Array(1D array=w153, element=w180) -> (index of element=w182:i32)  [unwired: 1 in]
                n268 = Search 1D Array(1D array=w153, element=w186) -> (index of element=w194:i32)  [unwired: 1 in]
                n269 = Search 1D Array(1D array=w153, element=w183) -> (index of element=w185:i32)  [unwired: 1 in]
                n270 = Search 1D Array(1D array=w153, element=w177) -> (index of element=w179:i32)  [unwired: 1 in]
                n271 = Search 1D Array(1D array=w153, element=w174) -> (index of element=w176:i32)  [unwired: 1 in]
                n272 = Search 1D Array(1D array=w153, element=w145) -> (index of element=w173:i32)  [unwired: 1 in]
                n273 = Concatenate Strings(w137, w155) -> (w154:string)
                n274 = Equal?(x=w182, y=-1) -> (x = y?=w170:bool)
                n275 = Equal?(x=w194, y=-1) -> (x = y?=w157:bool)
                n276 = Equal?(x=w185, y=-1) -> (x = y?=w171:bool)
                n277 = Equal?(x=w179, y=-1) -> (x = y?=w169:bool)
                n278 = Equal?(x=w176, y=-1) -> (x = y?=w168:bool)
                n279 = Equal?(x=w173, y=-1) -> (x = y?=w167:bool)
                n280 = Compound Arithmetic op=AND(w157, w171, w170, w169, w168, w167) -> ()  [unwired: 1 out]
                n281 = Search 1D Array(1D array=w153, element=w154) -> (index of element=w152:i32)  [unwired: 1 in]
                n282 = Index Array(array=w159, index=0) -> (element=w133:string)
                n283 = Equal?(x=w152, y=-1) -> (x = y?=w148:bool)
                n284 = And(x=w147, y=w148) -> (x .and. y?=w146:bool)
                n285 = case shown="True" w146 {
                  tunnel: w153 -> [_ w222]
                  tunnel: w137 -> [_ w218]
                  tunnel: [w214 w226] -> w143
                  tunnel: w166 -> [w214 w227]
                  tunnel: w156 -> [_ w216]
                  tunnel: w132 -> [w213 w221]
                  tunnel: [w213 w220] -> w131
                  frame False {
                  }
                  frame True {
                    n286 = local read "TAP"() -> (w217:string[][])
                    n287 = Index Array(array=w217, index (col)=0 ("disabled index (col)")) -> (element=w233:string[])  [unwired: 1 in]
                    n288 = Search 1D Array(1D array=w222, element="VACÍO") -> (index of element=w225:i32)  [unwired: 1 in]
                    n289 = Equal?(x=w225, y=-1) -> (x = y?=w223:bool)
                    n290 = Search 1D Array(1D array=w233, element=w218) -> (index of element=w228:i32)  [unwired: 1 in]
                    n291 = Increment(x=w216) -> (x+1=w229:enum8{"1", "2", "3", "4", "5", "6"})
                    n292 = case shown="\"1\", Default" w216 {
                      tunnel: [" a" " b" " c" " d" " e" " f"] -> w235
                      frame "1", Default {
                      }
                      frame "2" {
                      }
                      frame "3" {
                      }
                      frame "4" {
                      }
                      frame "5" {
                      }
                      frame "6" {
                      }
                    }
                    n293 = Concatenate Strings(w218, w235) -> (w219:string)
                    n294 = case shown="True" w223 {
                      tunnel: w222 -> [_ w251]
                      tunnel: w221 -> [w245 w253]
                      tunnel: [w245 w249] -> w220
                      tunnel: w219 -> [_ w252]
                      tunnel: w217 -> [w241 w246]
                      tunnel: w218 -> [w237 _]
                      tunnel: w216 -> [w240 _]
                      tunnel: [w238 w246] -> _
                      frame False {
                        n295 = Index Array(array=w241, index (col)=0 ("disabled index (col)")) -> (element=w243:string[])  [unwired: 1 in]
                        n296 = Search 1D Array(1D array=w243, element=w237) -> (index of element=w242:i32)  [unwired: 1 in]
                        n297 = Increment(x=w240) -> (x+1=w239:enum8{"1", "2", "3", "4", "5", "6"})
                        n298 = Replace Array Subset(array=w241, new element=w237, index (row)=w242, index (col)=w239) -> (w238:string[][])
                      }
                      frame True {
                        n299 = Equal?(x=w251, y="S.O.") -> (x = y?=w256:bool[])
                        n300 = Increment(x=w253) -> (x+1=w249:i16)
                        n301 = Boolean To (0,1)(Boolean=w256) -> (0, 1=w255:i16[])
                        n302 = Add Array Elements(numeric array=w255) -> (sum=w254:i16)
                        n303 = Increment(x=w254) -> (x+1=w250:i16)
                        "enum5" <- w250
                        n304 = Add(x=w250, y=w249) -> (x+y=w248:i16)
                        n305 = Replace Array Subset(array=w251, new element=w252, index=w248) -> (w247:string[])
                        n306 = local write "MemoryMap"(w247) -> ()
                      }
                    }
                    n307 = Replace Array Subset(array=w222, new element=w219, index=w225) -> (w232:string[])
                    n308 = local write "MemoryMap"(w232) -> ()
                    n309 = Search 1D Array(1D array=w232, element=w219) -> (index of element=w231:i32)  [unwired: 1 in]
                    n310 = Number To Decimal String(number=w231) -> (decimal integer string=w230:string)  [unwired: 1 in]
                    n311 = Replace Array Subset(array=w227, new element=w230, index (row)=w228, index (col)=w229) -> (w226:string[][])
                    n312 = Replace Array Subset(array=w217, new element=w230, index (row)=w228, index (col)=w229) -> (w215:string[][])
                    n313 = local write "TAP"(w215) -> ()
                  }
                }
                n314 = Index Array(array=w143, index (col)=0 ("disabled index (col)")) -> (element=w144:string[])  [unwired: 1 in]
                n315 = Search 1D Array(1D array=w144, element=w133) -> (index of element=w164:i32)  [unwired: 1 in]
                n316 = Search 1D Array(1D array=w144, element=w133) -> (index of element=w142:i32)  [unwired: 1 in]
                n317 = Index Array(array=w143, index (row)=w142) -> (element=w141:string[])  [unwired: 1 in]
                n318 = Index Array(array=w143, index (row)=w164, index (col)=1 ("disabled index (col)")) -> (element=w162:string)
                n319 = Equal?(x=w141, y="X") -> (x = y?=w139:bool[])
                n320 = Equal?(x=w162, y="D") -> (x = y?=w160:bool)
                n321 = case shown="False" w160 {
                  frame False {
                    n322 = local read "Enum 4"() -> (w202:enum8{"0", "1", "2", "3", "4", "5", "6"})
                    n323 = case shown="\"2\"" w202 {
                      tunnel: [u64 1 ("lower bound (0)") u64 2 ("upper bound (100)") u64 3 ("lower bound (0)") u64 4 ("lower bound (0)") u64 5 ("lower bound (0)") u64 6 ("lower bound (0)")] -> w204
                      frame "1", Default {
                      }
                      frame "2" {
                      }
                      frame "3" {
                      }
                      frame "4" {
                      }
                      frame "5" {
                      }
                      frame "6" {
                      }
                    }
                    n324 = call-poly <vilib>:"Random Number (Range).vi"("lower bound (0)"=u64 1, "upper bound (100)"=w204) -> ("number"=w203:u64)  [unwired: 9 in]
                    n325 = local write "Enum 3"(w203) -> ()
                  }
                  frame True {
                    n326 = local write "Enum 3"(enum16{"1", "2", "3", "4", "5", "6"}."1") -> ()
                  }
                }
                n327 = Boolean To (0,1)(Boolean=w139) -> (0, 1=w138:i16[])
                n328 = Add Array Elements(numeric array=w138) -> (sum=w136:i16)
                "sum" <- w136
                n329 = Subtract(x=i16 6, y=w136) -> (x-y=w134:i16)
                n330 = local write "Enum 4"(w134) -> ()
              }
            }
            n331 = local read "element"() -> (w72:string)
            n332 = Equal?(x=w73, y=w72) -> (x = y?=w71:bool)
            n333 = Not(x=w71) -> (.not. x?=w70:bool)
            n334 = And(x=w62, y=w70) -> (x .and. y?=w69:bool)
            n335 = case shown="True" w69 {
              tunnel: w74 -> [_ w274]
              tunnel: w75 -> [w270 w273]
              tunnel: [w270 w272] -> w47
              tunnel: w72 -> [_ w271]
              frame False {
              }
              frame True {
                n336 = Insert Into Array(array=w273, index=w274, new element=w271) -> (w272:string[])
              }
            }
            n337 = local write "Printing 2"(w46) -> ()
            n338 = local write "Waiting 2"(w44) -> ()
            n339 = local write "Ready"(w47) -> ()
            n340 = Equal?(x=i64 3, y=w49) -> (x = y?=w56:bool)
            n341 = local write "Waiting 2"(w61) -> ()
            n342 = local write "TAP 2"(w51) -> ()
            n343 = case shown="True" w56 {
              tunnel: w49 -> [w120 w127]
              tunnel: [w120 w125] -> w48
              tunnel: w47 -> [w119 w124]
              tunnel: w46 -> [_ w122]
              tunnel: [w119 w121] -> w45
              frame False {
              }
              frame True {
                n344 = invoke on="Printing 2" class="Str" method="Reinit To Default"() -> ()  [unwired: 3 in, 3 out]
                n345 = Array Size(array=w124) -> (size(s)=w123:i32)
                n346 = Subtract(x=w127, y=i64 3) -> (x-y=w125:i64)
                n347 = Insert Into Array(array=w124, index=w123, new element=w122) -> (w121:string[])
              }
            }
            n348 = local write "Ready"(w45) -> ()
          }
        }
        n349 = case shown="True" "play/pause" {
          frame False {
          }
          frame True {
            n350 = while {
              stop <- w525 continue-if-true
              n351 = local read "play/pause"() -> (w525:bool)
              n352 = Wait (ms)(milliseconds to wait=u32 10) -> ()  [unwired: 1 out]
            }
          }
        }
        n353 = call "Display Message to User"("Enable"="stop") -> ("SÍ"=w25:bool)  [unwired: 9 in, 1 out]
        n354 = Wait (ms)(milliseconds to wait="Delay") -> ()  [unwired: 1 out]
        "Clock" <- w22
      }
    }
  }
